vi "Test Error If Mock Not Initialized.vi"(8 "error in (no error)":errorcluster, 11 "Expectation Test in":refnum<class "Expectation Test.lvclass">) -> (0 "error out":errorcluster, 3 "Expectation Test out":refnum<class "Expectation Test.lvclass">)   [LabVIEW 2020, in "Expectation Test.lvclass"]
uses:
  Expectation Test.lvclass
  C:/Program Files (x86)/National Instruments/LabVIEW 2020/vi.lib/Astemes/LUnit/Test Case.lvclass
  <vilib>/Astemes/LUnit/Test Case.lvclass
  source/Framework/Mock/LMock Mock.lvclass
  <vilib>/Astemes/LUnit/Test Case.lvclass/Test Case.ctl
  <vilib>/Astemes/LUnit/Append Fail Result.vi
  <vilib>/Astemes/LUnit/Append Pass Result.vi
  source/Framework/Verifier/Verifier.lvclass
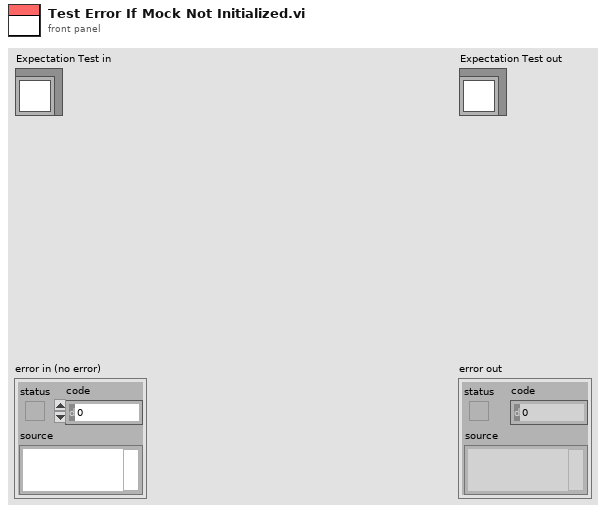
[diagram p1: front panel]
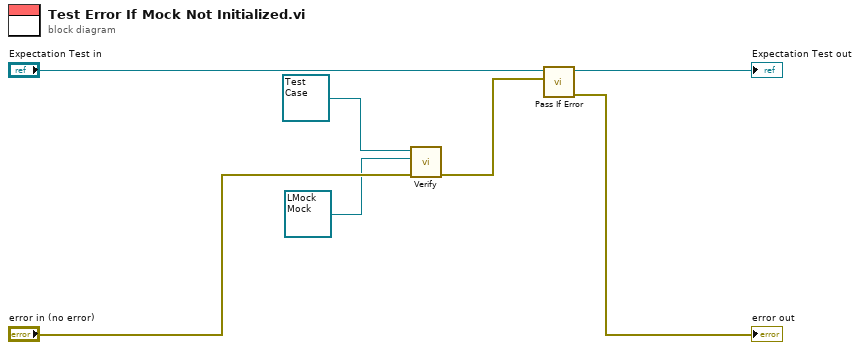
[diagram p0: block diagram]
diagram:
  n1 = call "Verify.vi"("error in (no error)"="error in (no error)", "Mock"=refnum<class "LMock Mock.lvclass"> refnum, "LUnit Test Case In"=refnum<class "Test Case.lvclass"> refnum) -> ("error out"=w1:errorcluster)  [unwired: 7 in, 1 out]
  n2 = call <vilib>:"Pass If Error.vi"("Assert error"=w1, "LUnit Test Case In"="Expectation Test in") -> ("error out"=→"error out":errorcluster, "LUnit Test Case Out"=→"Expectation Test out":refnum<class "Expectation Test.lvclass">)  [unwired: 8 in]
